vi "State_history.vi"(11 "element":T1) -> (3 "Array":T1[](array[typedef]))   [LabVIEW 2018]
uses:
  controls/Control RT Code.ctl
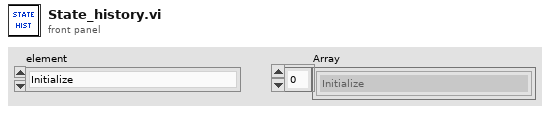
[diagram p1: front panel]
types:
  T1 = typedef "Control RT Code.ctl" = enum16{"Initialize", "Start New Test", "Stop Trial", "Start New Trial", "Load Trial Config Settings", "Load Rig Config Settings", "Determine Which Trial to Run", "Download All Trials to RT System", "Create New Folder", "Create New Data File", "Inter-Trial Interval Delay", "Initialize Trial Tracker", "Update Water Tracker", "Update Trial Tracker", "Exit"}
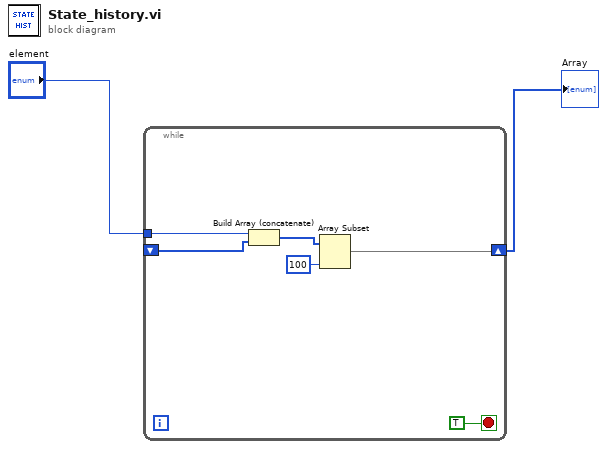
[diagram p0: block diagram]
diagram:
  n1 = while {
    shift-right: [w3] -> w1
    shift-left: _ -> [w6]
    tunnel: "element" -> [w7]
    stop <- TRUE stop-if-true
    n2 = Build Array (concatenate)(w7, w6) -> (w5:T1[])
    n3 = Array Subset(array=w5, length=100) -> (w3:T1[])  [unwired: 1 in]
  }
  "Array" <- w1
